vi "pcfs_get_duration.vi"(5 "total_steps":u32, 7 "current_iteration":u32, 8 "error in (no error)":errorcluster, 10 "current_position":dbl, 11 "scan_panel in":refnum<class "pcfs.lvclass">) -> (0 "error out":errorcluster, 2 "time_remaining":string, 3 "scan_panel out":refnum<class "pcfs.lvclass">)   [LabVIEW 2015, in "pcfs.lvclass"]
uses:
  pcfs.lvclass
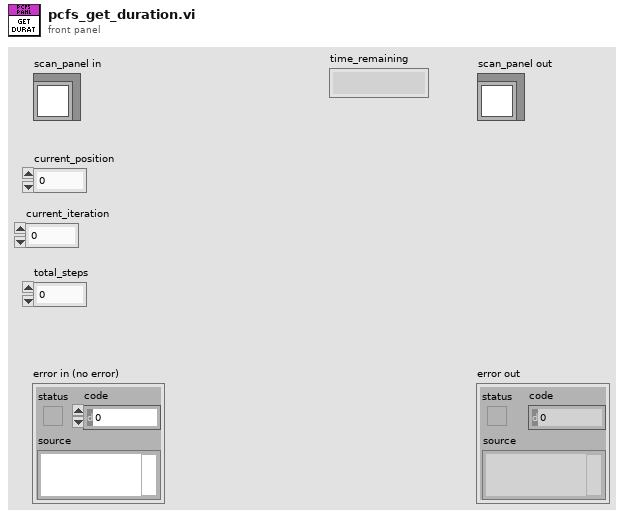
[diagram p1: front panel]
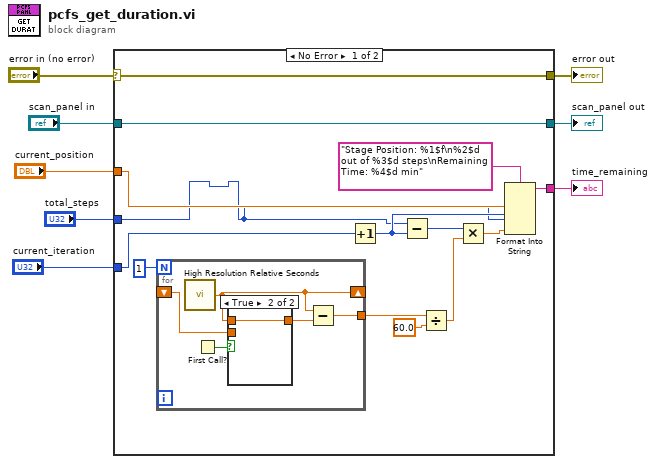
[diagram p0: block diagram]
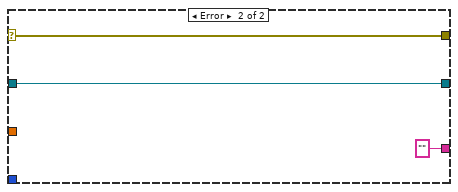
[diagram p3: hidden frame]
diagram:
  n1 = case shown="No Error" "error in (no error)" {
    selector: "error in (no error)" -> [w21 w32]
    tunnel: [w21 w32] -> w7
    tunnel: [w22 w31] -> w5
    tunnel: "scan_panel in" -> [w22 w31]
    tunnel: "current_position" -> [w19 _]
    tunnel: "current_iteration" -> [w11 _]
    tunnel: "total_steps" -> [w9 _]
    tunnel: [w12 ""] -> w1
    frame No Error {
      n2 = for {
        N: 1 -> [_]
        shift-right: [w24] -> _
        shift-left: _ -> [w26]
        tunnel: [w27] -> w17
        n3 = call <vilib>:"High Resolution Relative Seconds.vi"() -> ("relative seconds"=w24:dbl)
        n4 = First Call?() -> (First Call?: T/F=w23:bool)
        n5 = case shown="True" w23 {
          tunnel: w26 -> [w28 _]
          tunnel: [w28 w29] -> w25
          tunnel: w24 -> [_ w29]
          frame False {
          }
          frame True {
          }
        }
        n6 = Subtract(x=w24, y=w25) -> (x-y=w27:dbl)
      }
      n7 = Increment(x=w11) -> (x+1=w10:u32)
      n8 = Subtract(x=w9, y=w10) -> (x-y=w15:u32)
      n9 = Divide(x=w17, y=60.0) -> (x/y=w14:dbl)
      n10 = Multiply(x=w15, y=w14) -> (x*y=w13:dbl)
      n11 = Format Into String(format string="Stage Position: %1$f\n%2$d out of %3$d steps\nRemaining Time: %4$d min", w19, w10, w9, w13) -> (resulting string=w12:string)  [unwired: 2 in, 1 out]
    }
    frame Error {
    }
  }
  "error out" <- w7
  "scan_panel out" <- w5
  "time_remaining" <- w1
